vi "main-vi.vi"(1 "Enable":bool) -> ()   [LabVIEW 2017]
panel:
  in  "Stop":bool
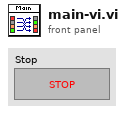
[diagram p1: front panel]
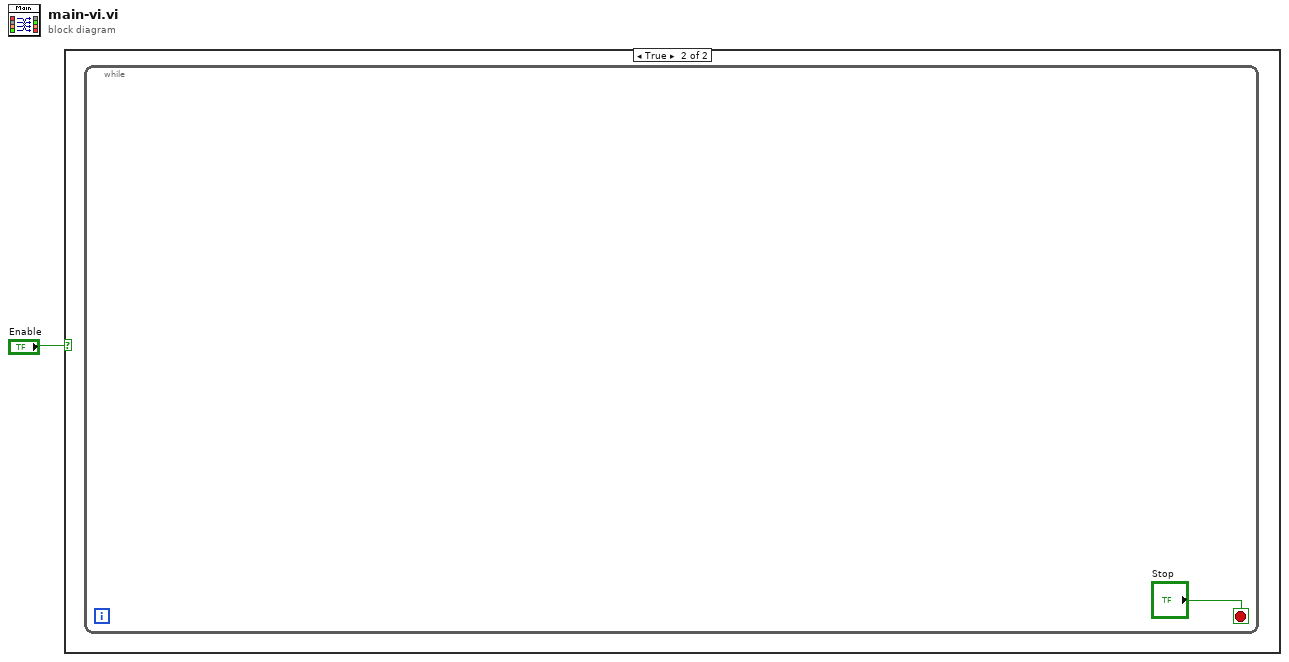
[diagram p0: block diagram]
diagram:
  n1 = case shown="True" "Enable" {
    frame False {
    }
    frame True {
      n2 = while {
        stop <- "Stop" stop-if-true
      }
    }
  }
